vi "Handle setAllData.vi"(8 "error in (no error)":errorcluster, 10 "AllData":variant, 11 "Inst.Transport in":refnum<class "Inst.Transport.lvclass">) -> (0 "error out":errorcluster, 3 "Inst.Transport out":refnum<class "Inst.Transport.lvclass">)   [LabVIEW 2019, in "Inst.Transport.lvclass"]
doc: "Override to handle \"getAll\" or \"getAllData\" commands for <b>your</b> Instrument"
uses:
  Inst.Transport.lvclass
  Inst.Transport.lvclass/Inst.Transport.ctl
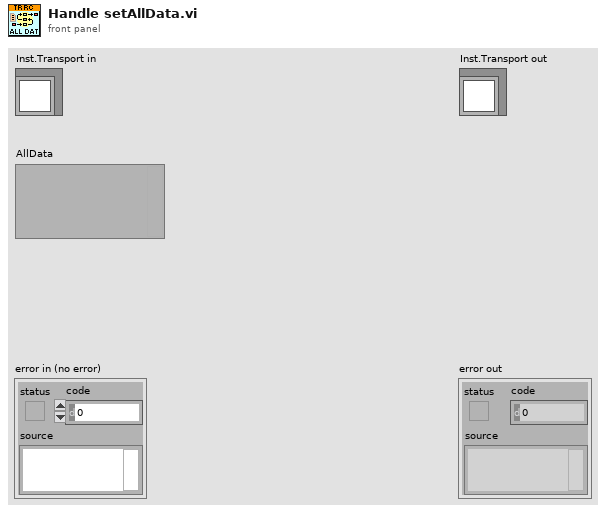
[diagram p1: front panel]
types:
  T1 = typedef "Inst.Transport.lvclass/Inst.Transport.getAll--Cluster.ctl" = cluster{"data":variant}
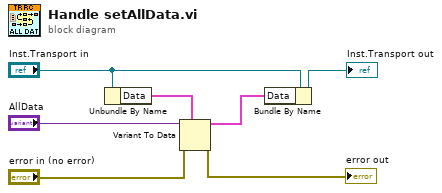
[diagram p0: block diagram]
diagram:
  n1 = Unbundle By Name("Inst.Transport in") -> ("Data"=w5:T1)
  n2 = Variant To Data(error in="error in (no error)", type=w5, Variant="AllData") -> (data=w3:T1, error out=→"error out":errorcluster)
  n3 = Bundle By Name(cluster="Inst.Transport in", "Data"=w3) -> (→"Inst.Transport out":refnum<class "Inst.Transport.lvclass">)
